vi "Get Last Reading.vi"(8 "error in":errorcluster, 10 "Channel":string, 11 "BufferLastReadingsDBL in":refnum<class "BufferLastReadsDBL.lvclass">) -> (0 "error out":errorcluster, 2 "Reading":dbl, 3 "BufferLastReadingsDBL out":refnum<class "BufferLastReadsDBL.lvclass">)   [LabVIEW 2023, in "BufferLastReadsDBL.lvclass"]
uses:
  BufferLastReadsDBL.lvclass
  BufferLastReadsDBL.lvclass/BufferLastReadsDBL.ctl
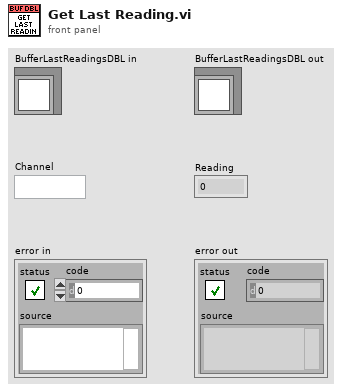
[diagram p1: front panel]
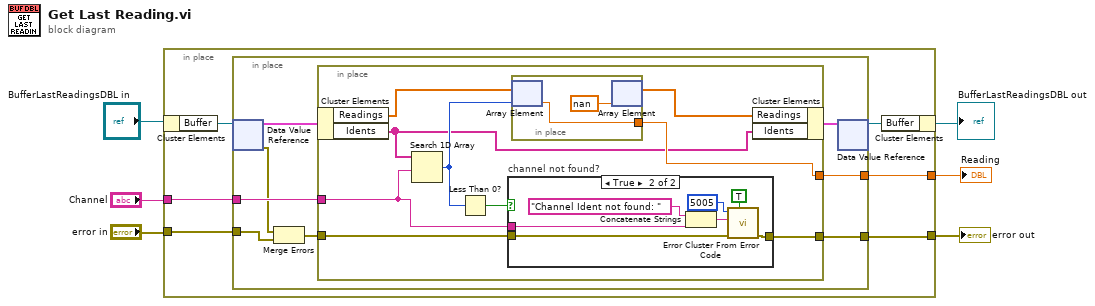
[diagram p0: block diagram]
diagram:
  n1 = in-place {
    in-place-border: "Channel" -> [w11]
    in-place-border: "error in" -> [w10]
    in-place-border: [w7] -> w4
    in-place-border: [w8] -> w1
    n2 = in-place-cluster #1("BufferLastReadingsDBL in") -> ("Buffer"=w12:refnum<data-value>)
    n3 = in-place {
      in-place-border: w11 -> [w17]
      in-place-border: w10 -> [w20]
      in-place-border: [w19] -> w8
      in-place-border: [w18] -> w7
      n4 = in-place-dvr #2(w12) -> (w14:cluster{"Idents":string[], "Readings":dbl[]}, w15:errorcluster)
      n5 = Merge Errors(w15, w20) -> (w16:errorcluster)
      n6 = in-place {
        in-place-border: [w22] -> w19
        in-place-border: [w29] -> w18
        in-place-border: w17 -> [w28]
        in-place-border: w16 -> [w25]
        n7 = in-place-cluster #3(w14) -> ("Readings"=w24:dbl[], "Idents"=w21:string[])
        n8 = Search 1D Array(1D array=w21, element=w28) -> (index of element=w26:i32)  [unwired: 1 in]
        n9 = Less Than 0?(x=w26) -> (x < 0?=w27:bool)
        n10 = case "channel not found?" shown="True" w27 {
          tunnel: [w30 w34] -> w29
          tunnel: w25 -> [w30 w33]
          tunnel: w28 -> [_ w32]
          frame False {
          }
          frame True {
            n11 = Concatenate Strings("Channel Ident not found: " ("error message (\"\")"), w32) -> (w36:string)
            n12 = call <vilib>:"Error Cluster From Error Code.vi"("show call chain? (False)"=TRUE, "error in (no error)"=w33, "error message (\"\")"=w36, "error code (0)"=5005) -> ("error out"=w34:errorcluster)  [unwired: 5 in]
          }
        }
        n13 = in-place {
          in-place-border: [w38] -> w22
          n14 = in-place-array #4(w24, w26) -> (w38:dbl)
          n15 = in-place-array #4(nan) -> (w23:dbl[])  [unwired: 1 out]
        }
        n16 = in-place-cluster #3("Readings"=w23, "Idents"=w21) -> (w13:cluster{"Idents":string[], "Readings":dbl[]})
      }
      n17 = in-place-dvr #2(w13) -> (w9:refnum<data-value>)  [unwired: 1 out]
    }
    n18 = in-place-cluster #1("Buffer"=w9) -> (→"BufferLastReadingsDBL out":refnum<class "BufferLastReadsDBL.lvclass">)
  }
  "error out" <- w4
  "Reading" <- w1
